vi "get ListenerID.vi"(0 "Session Handle in":T1, 11 "error in (no error)":errorcluster) -> (4 "Session Handle out":T1, 6 "Session Name":string, 15 "error out":errorcluster)   [LabVIEW 2012, in "REx.lvlib" / "Local Listener Session.lvclass"]
uses:
  Local Listener Session.lvclass
  Typedefs/Session Handle.ctl
  Local Listener Session.lvclass/Local Listener Session.ctl
  <userlib>/_Session Fwk/Session - Root.lvclass
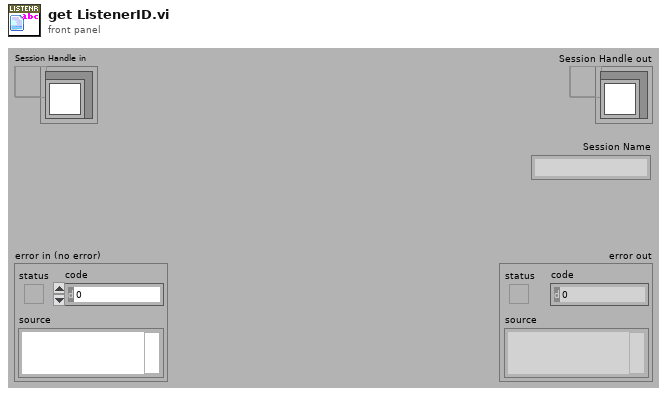
[diagram p1: front panel]
types:
  T1 = typedef "REx.lvlib/Local Listener Session.lvclass/Session Handle.ctl" = refnum<data-value>
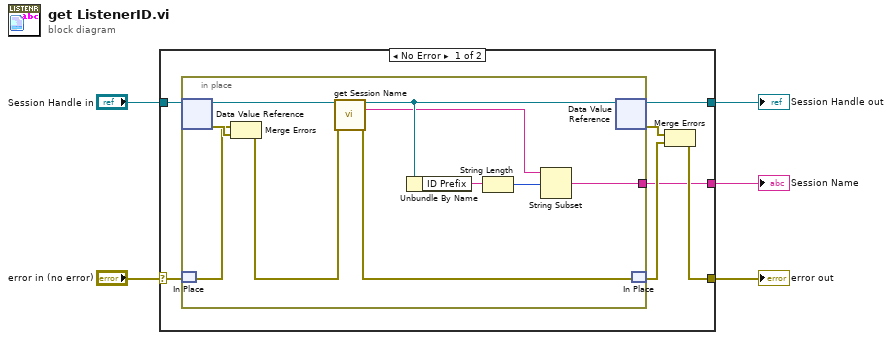
[diagram p0: block diagram]
diagram:
  n1 = case shown="No Error" "error in (no error)" {
    selector: "error in (no error)" -> [w7 w23]
    tunnel: "Session Handle in" -> [w12 w24]
    tunnel: [w11 w24] -> w4
    tunnel: [w8 w23] -> w3
    tunnel: [w6 _] -> w1
    frame No Error {
      n2 = in-place {
        in-place-border: [w14] -> w6
        n3 = in-place-dvr #1(w12) -> (w20:refnum<class "Local Listener Session.lvclass">, w22:errorcluster)
        n4 = in-place-match #2(w7) -> (w21:errorcluster)
        n5 = Merge Errors(w21, w22) -> (w19:errorcluster)
        n6 = call <userlib>:"get Session Name.vi"("OBJ - Session in"=w20, "error in (no error)"=w19) -> ("OBJ - Session out"=w17:refnum<class "Local Listener Session.lvclass">, "Session Name"=w13:string, "error out"=w18:errorcluster)  [unwired: 11 in]
        n7 = Unbundle By Name(w17) -> ("ID Prefix"=w16:string)
        n8 = String Length(string=w16) -> (length=w15:i32)
        n9 = String Subset(string=w13, offset (0)=w15) -> (substring=w14:string)  [unwired: 1 in]
        n10 = in-place-dvr #1(w17) -> (w11:T1, w9:errorcluster)
        n11 = in-place-match #2(w18) -> (w10:errorcluster)
      }
      n12 = Merge Errors(w9, w10) -> (w8:errorcluster)
    }
    frame Error {
    }
  }
  "Session Handle out" <- w4
  "error out" <- w3
  "Session Name" <- w1
